vi "Battery Emulated.vi"() -> ()   [LabVIEW 2018]
uses:
  <instrlib>/niDCPower/nidcpower.llb/niDCPower Wait For Event - Event.ctl
  <instrlib>/niDCPower/nidcpower.llb/niDCPower Source Mode.ctl
  <instrlib>/niDCPower/nidcpower.llb/niDCPower Output Function.ctl
panel:
  out "Waveform Chart":cluster{dbl, dbl}(graph)
  in  "stop":bool
  in  "voltage level":dbl caption="Battery Voltage" format="%.6p"
  in  "Internal Resistance of Battery":dbl
  in  "Source Delay (Sec)":dbl=0.005
  in  "Current Limit":dbl=0.01
  in  "Channel Name":string="0"
  in  "Resource Name":refnum<k15>="Dev1"
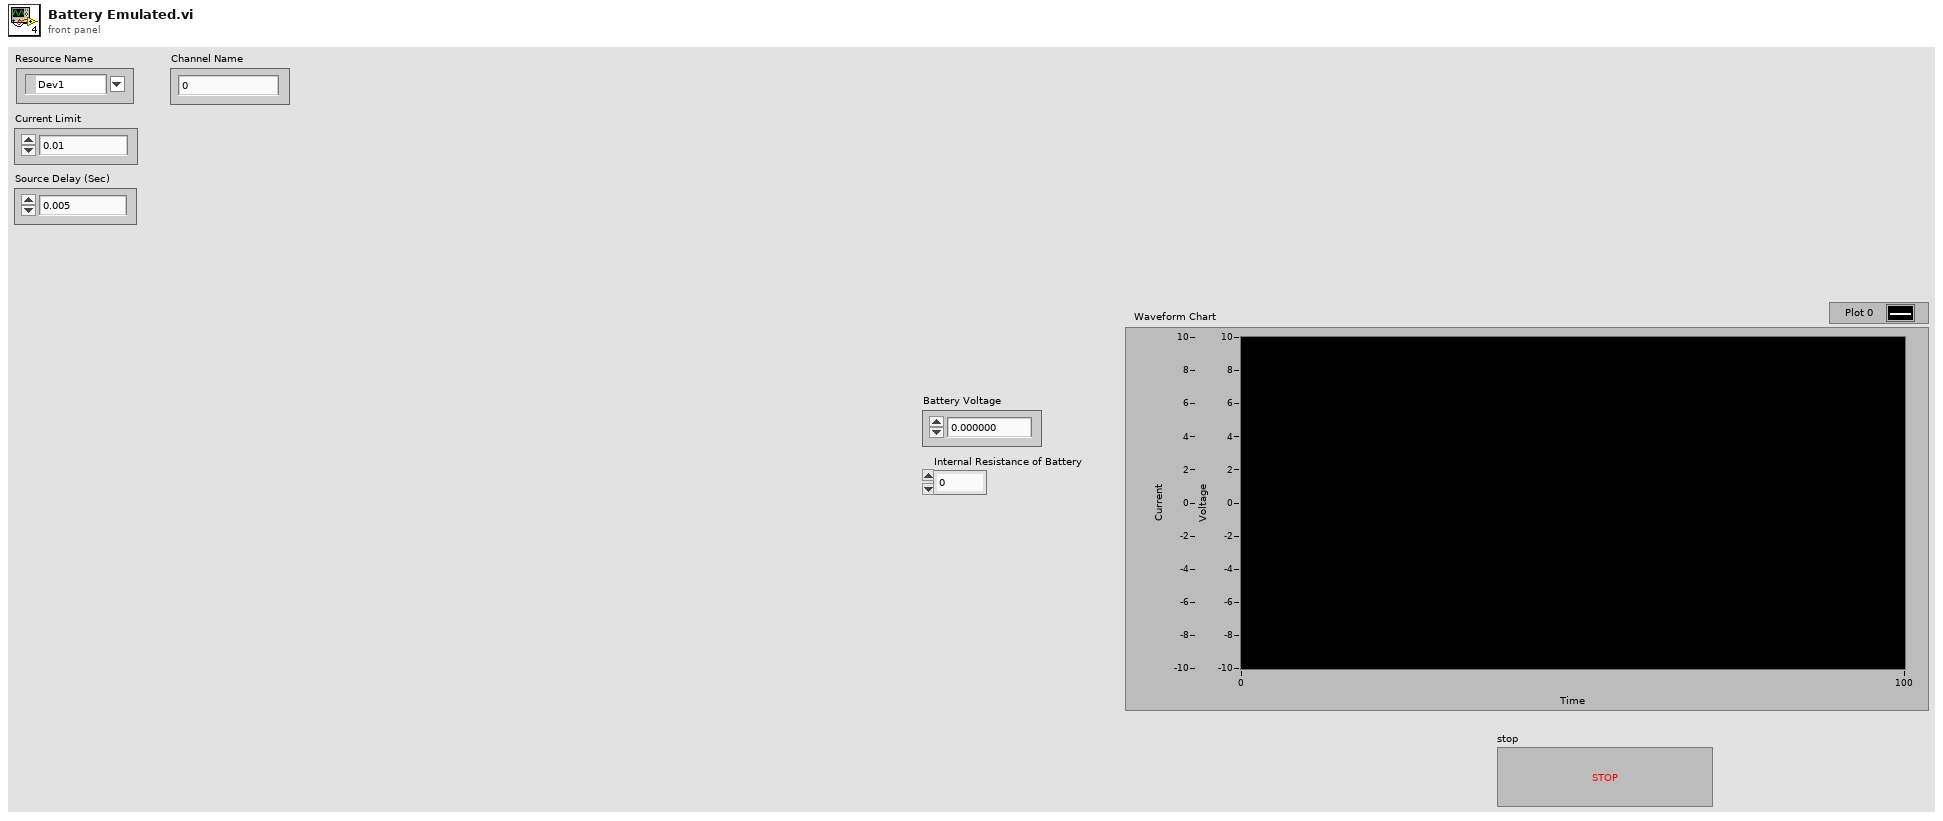
[diagram p1: front panel]
types:
  T1 = typedef "niDCPower Output Function.ctl" = i32
  T2 = typedef "niDCPower Source Mode.ctl" = i32
  T3 = typedef "niDCPower Wait For Event - Event.ctl" = i32
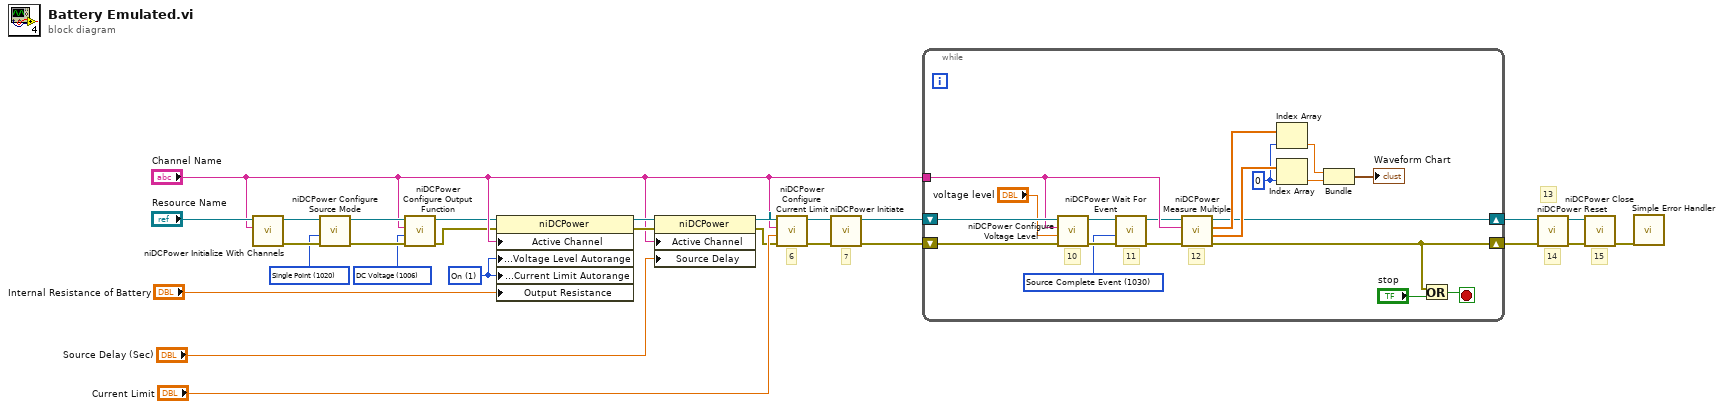
[diagram p0: block diagram]
diagram:
  w4 = T1 1006 items=["DC Voltage"=1006, "DC Current"=1007, "Pulse Voltage"=1049, "Pulse Current"=1050] ("output function")
  w14 = T2 1020 items=["Single Point"=1020, "Sequence"=1021] ("source mode")
  w5 = 1 items=["Off", "On"] ("DC Voltage:Voltage Level Autorange")
  # "6"
  # "13"
  # "15"
  # "14"
  # "7"
  n1 = call <instrlib>:"niDCPower Initialize With Channels.vi"("channels"="Channel Name", "resource name"="Resource Name") -> ("error out"=w18:errorcluster, "instrument handle out"=w16:refnum<k15>)  [unwired: 3 in, 5 out]
  n2 = call <instrlib>:"niDCPower Configure Source Mode.vi"("error in (no error)"=w18, "source mode"=w14, "instrument handle"=w16) -> ("error out"=w17:errorcluster, "instrument handle out"=w15:refnum<k15>)  [unwired: 7 out]
  n3 = call <instrlib>:"niDCPower Configure Output Function.vi"("error in (no error)"=w17, "output function"=w4, "channel name"="Channel Name", "instrument handle"=w15) -> ("error out"=w6:errorcluster, "instrument handle out"=w7:refnum<k15>)  [unwired: 6 out]
  n4 = property class="niDCPower"(reference=w7, error in=w6, "Active Channel"="Channel Name", "Source:DC Voltage:Voltage Level Autorange"=w5, "Source:DC Voltage:Current Limit Autorange"=w5, "Output Resistance"="Internal Resistance of Battery") -> (reference out=w13:refnum<k15>, error out=w10:errorcluster)
  n5 = property class="niDCPower"(reference=w13, error in=w10, "Active Channel"="Channel Name", "Source Delay"="Source Delay (Sec)") -> (reference out=w12:refnum<k15>, error out=w11:errorcluster)
  n6 = call <instrlib>:"niDCPower Configure Current Limit.vi"("error in (no error)"=w11, "current limit"="Current Limit", "channel name"="Channel Name", "instrument handle"=w12) -> ("error out"=w1:errorcluster, "instrument handle out"=w2:refnum<k15>)  [unwired: 6 out]
  n7 = call <instrlib>:"niDCPower Initiate.vi"("error in (no error)"=w1, "instrument handle"=w2) -> ("error out"=w21:errorcluster, "instrument handle out"=w22:refnum<k15>)  [unwired: 8 out]
  n8 = while {
    shift-right: [w31] -> w19
    shift-left: w21 -> [w45]
    shift-right: [w39] -> w20
    shift-left: w22 -> [w46]
    tunnel: "Channel Name" -> [w44]
    stop <- w29 stop-if-true
    w34 = T3 1030 items=["Source Complete Event"=1030, "Measure Complete Event"=1031, "Sequence Iteration Complete Event"=1032, "Sequence Engine Done Event"=1033] ("event")
    w33 = 0 ("index")
    # "11"
    # "12"
    # "10"
    n9 = call <instrlib>:"niDCPower Configure Voltage Level.vi"("error in (no error)"=w45, "voltage level"="voltage level", "channel name"=w44, "instrument handle"=w46) -> ("error out"=w38:errorcluster, "instrument handle out"=w35:refnum<k15>)  [unwired: 6 out]
    n10 = call <instrlib>:"niDCPower Wait For Event.vi"("error in (no error)"=w38, "event"=w34, "instrument handle"=w35) -> ("error out"=w37:errorcluster, "instrument handle out"=w36:refnum<k15>)  [unwired: 1 in, 6 out]
    n11 = call <instrlib>:"niDCPower Measure Multiple.vi"("error in (no error)"=w37, "channel name"=w44, "instrument handle"=w36) -> ("error out"=w31:errorcluster, "current measurements"=w43:dbl[], "voltage measurements"=w42:dbl[], "instrument handle out"=w39:refnum<k15>)  [unwired: 5 out]
    n12 = Index Array(array=w42, index=w33) -> (element=w41:dbl)
    n13 = Index Array(array=w43, index=w33) -> (element=w40:dbl)
    n14 = Bundle(w41, w40) -> (→"Waveform Chart":cluster{dbl, dbl})  [unwired: 1 out]
    n15 = Or(x=w31, y="stop") -> (x .or. y?=w29:bool)
  }
  n16 = call <instrlib>:"niDCPower Reset.vi"("error in (no error)"=w19, "instrument handle"=w20) -> ("error out"=w26:errorcluster, "instrument handle out"=w25:refnum<k15>)  [unwired: 8 out]
  n17 = call <instrlib>:"niDCPower Close.vi"("error in (no error)"=w26, "instrument handle"=w25) -> ("error out"=w24:errorcluster)  [unwired: 9 out]
  n18 = call <vilib>:"Simple Error Handler.vi"("error in (no error)"=w24) -> ()  [unwired: 1 in, 8 out]
